vi "Dipper Fridge Resistance Measurement 2.0.vi"() -> ()   [LabVIEW 2011]
panel:
  in  "Lower critical\ntemperature":dbl
  in  "Upper critical\ntemperature":dbl
  out "x > y?":bool
  in  "critical temperature\n time delay":dbl
  out "error out":errorcluster
  in  "error in (no error)":errorcluster
  out "appended array 3":dbl[](array[numeric])
  out "appended array 2":dbl[](array[numeric])
  in  "General time delay":dbl
  out "appended array":dbl[](array[numeric])
  out "Temperature Vs Time":cluster{dbl[], dbl[]}(graph)
  out "Current Resistance":string
  in  "error in (no error) 3":errorcluster
  out "Current Temperature":string
  in  "Heater option":string
  out "Sample Vs. Temp":cluster{dbl[], dbl[]}(graph)
  out "Warning":string="Can't be smaller than 1 s"
  in  "Timer":bool caption="Reset"
  out "Time Elapsed":string
  in  "Save":bool
  out "var":i32
  out "Heater":bool
  in  "Heater":bool
  out "Boolean":bool
  in  "Power":bool
  in  "Date format (0)":enum16{"short", "long", "abbreviated"}(ring)
  in  "File Path":path
  out "current time":timestamp
  out "Data points":i32
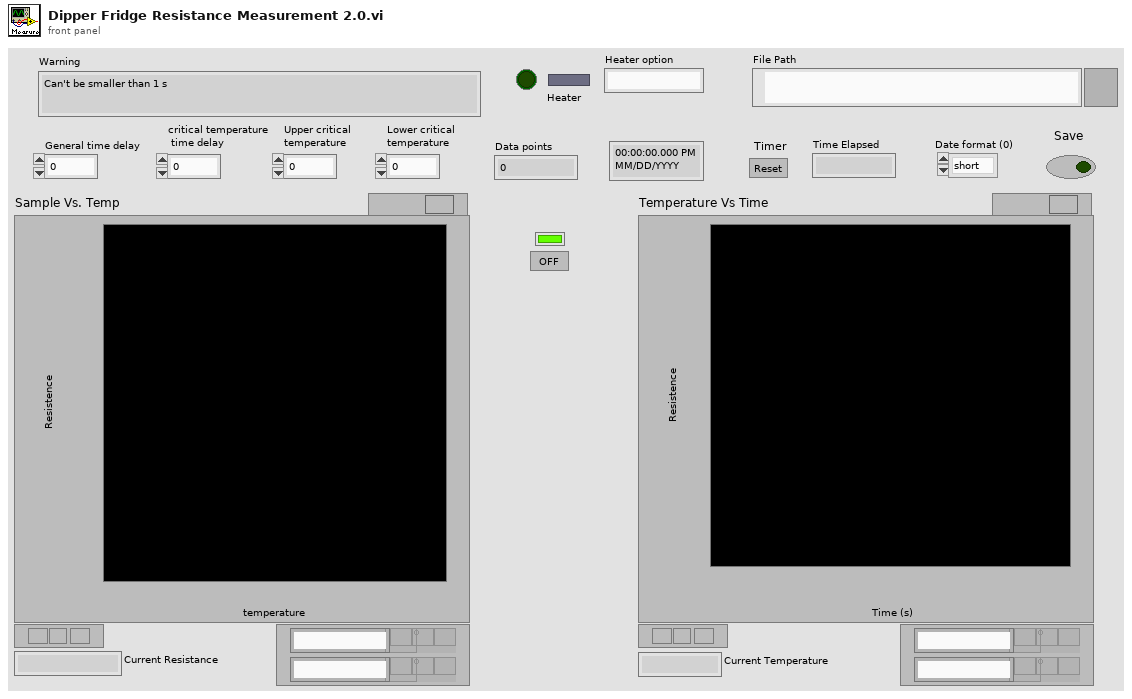
[diagram p1: front panel]
types:
  T1 = enum16{"open", "replace", "create", "open or create", "replace or create", "replace or create with confirmation"}
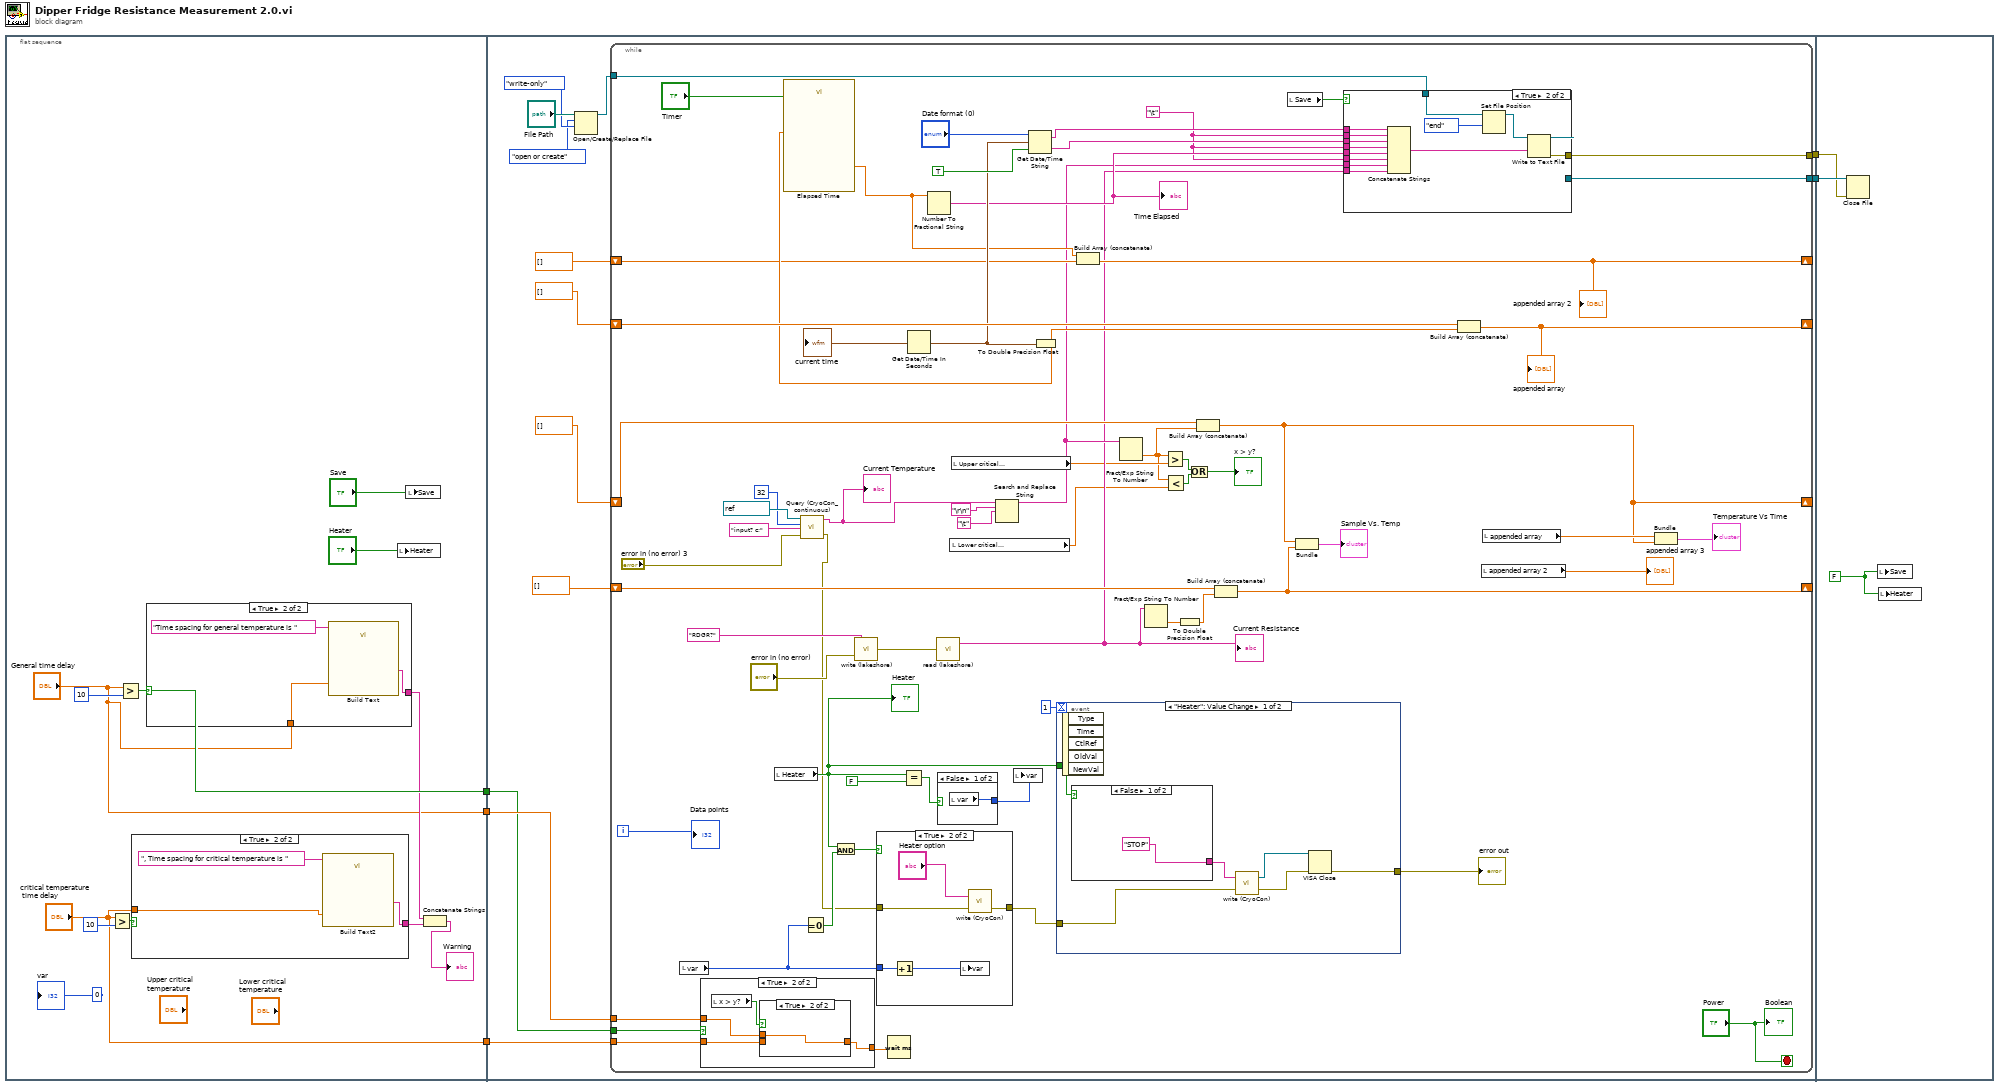
[diagram p0: block diagram]
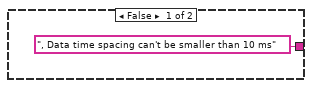
[diagram p2: hidden frame]
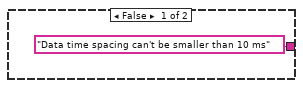
[diagram p3: hidden frame]
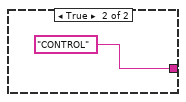
[diagram p4: hidden frame]
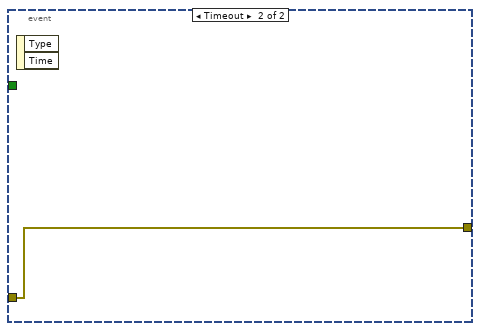
[diagram p5: hidden frame]
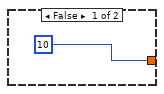
[diagram p6: hidden frame]
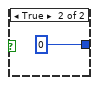
[diagram p8: hidden frame]
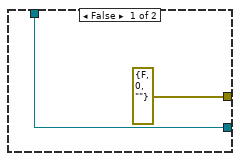
[diagram p10: hidden frame]
diagram:
  n1 = flat-sequence {
    tunnel: ["General time delay"] -> w5
    tunnel: [w13] -> w4
    tunnel: ["critical temperature\n time delay"] -> w1
    tunnel: w5 -> [w35]
    tunnel: w4 -> [w34]
    tunnel: [w28] -> w3
    tunnel: [w27] -> w2
    tunnel: w1 -> [w26]
    tunnel: w3 -> [w143]
    tunnel: w2 -> [w142]
    frame #0 {
      n2 = Greater?(x="critical temperature\n time delay", y=u32 10 ("x")) -> (0:w11:bool)
      n3 = Greater?(x="General time delay", y=u32 10 ("x")) -> (0:w13:bool)
      n4 = case shown="True" w11 {
        tunnel: [", Data time spacing can't be smaller than 10 ms" w21] -> w10
        tunnel: "critical temperature\n time delay" -> [_ w20]
        frame False {
        }
        frame True {
          n5 = call "Build Text2"("Beginning Text"=", Time spacing for critical temperature is ", "Y"=w20) -> ("Result"=w21:string)  [unwired: 12 in, 1 out]
        }
      }
      n6 = case shown="True" w13 {
        tunnel: "General time delay" -> [_ w24]
        tunnel: ["Data time spacing can't be smaller than 10 ms" w23] -> w9
        frame False {
        }
        frame True {
          n7 = call "Build Text"("Beginning Text"="Time spacing for general temperature is ", "Y"=w24) -> ("Result"=w23:string)  [unwired: 12 in, 1 out]
        }
      }
      n8 = local write "Heater"("Heater") -> ()
      n9 = local write "Save"("Save") -> ()
      n10 = Concatenate Strings(w9, w10) -> (→"Warning":string)
      "var" <- 0 ("var")
    }
    frame #1 {
      n11 = Open/Create/Replace File(file path (use dialog)="File Path", operation (0:open)=T1."open or create", access (0:read/write)=enum16{"read/write", "read-only", "write-only"}."write-only") -> (refnum out=w31:refnum<file>)  [unwired: 3 in, 2 out]
      n12 = while {
        shift-right: [w79] -> _
        shift-left: dbl[] [] -> [w99]
        shift-right: [w67] -> _
        shift-left: dbl[] [] -> [w97]
        shift-right: [w78] -> _
        shift-left: dbl[] [] -> [w83]
        tunnel: w35 -> [w80]
        tunnel: w34 -> [w81]
        shift-right: [w75] -> _
        shift-left: dbl[] [] -> [w76]
        tunnel: w31 -> [w54]
        tunnel: [w53] -> w28
        tunnel: [w52] -> w27
        tunnel: w26 -> [w45]
        i -> [w101]
        stop <- "Power" stop-if-true
        w57 = "\t"
        n13 = local read "var"() -> (w95:i32)
        n14 = case shown="True" w81 {
          tunnel: [10 w114] -> w82
          tunnel: w80 -> [_ w115]
          tunnel: w45 -> [_ w113]
          frame False {
          }
          frame True {
            n15 = local read "x > y?"() -> (w112:bool)
            n16 = case shown="True" w112 {
              tunnel: [w116 w117] -> w114
              tunnel: w115 -> [_ w117]
              tunnel: w113 -> [w116 _]
              frame False {
              }
              frame True {
              }
            }
          }
        }
        n17 = local read "Heater"() -> (w87:bool)
        "Heater" <- w87
        n18 = call "Query (CryoCon_continuous).vi"("error in (no error)"="error in (no error) 3", "write buffer"="input? c;", "byte count"=u32 32, "VISA resource name"=refnum<visa-resource-name> "COM3" ("VISA resource name 2")) -> ("error out"=w50:errorcluster, "read buffer"=w51:string)  [unwired: 1 out]
        "Current Temperature" <- w51
        n19 = Equal To 0?(x=w95) -> (x = 0?=w94:bool)
        n20 = And(x=w87, y=w94) -> (x .and. y?=w93:bool)
        n21 = call "write (lakeshore).vi"("error in (no error)"="error in (no error)", "write buffer"="RDGR?") -> ("error out"=w71:errorcluster)
        n22 = case shown="True" w93 {
          tunnel: [w120 w124] -> w92
          tunnel: w95 -> [_ w122]
          tunnel: w50 -> [w120 w123]
          frame False {
          }
          frame True {
            n23 = Increment(x=w122) -> (x+1=w121:i32)
            n24 = local write "var"(w121) -> ()
            n25 = call "write (CryoCon).vi"("error in (no error)"=w123, "write buffer"="Heater option") -> ("error out"=w124:errorcluster)  [unwired: 1 out]
          }
        }
        n26 = Wait (ms)(milliseconds to wait=w82) -> ()  [unwired: 1 out]
        n27 = Equal?(x=w87, y=FALSE ("Heater")) -> (x = y?=w89:bool)
        n28 = Get Date/Time In Seconds() -> (seconds since 1Jan1904=w86:timestamp)
        "current time" <- w86
        n29 = call "read (lakeshore).vi"("error in (no error)"=w71) -> ("read buffer"=w55:string)  [unwired: 1 out]
        "Current Resistance" <- w55
        n30 = case shown="False" w89 {
          tunnel: [w118 0] -> w88
          frame False {
            n31 = local read "var"() -> (w118:i32)
          }
          frame True {
          }
        }
        n32 = local read "Lower critical\ntemperature"() -> (w42:dbl)
        n33 = local read "Upper critical\ntemperature"() -> (w44:dbl)
        n34 = Search and Replace String(input string=w51, search string="\r\n", replace string="\t") -> (result string=w56:string)  [unwired: 5 in, 3 out]
        n35 = local write "var"(w88) -> ()
        n36 = Get Date/Time String(date format (0)="Date format (0)", seconds (now)=w86, want seconds? (F)=TRUE) -> (date string=w60:string, time string=w59:string)
        n37 = To Double Precision Float(number=w86) -> (double precision float=w85:dbl)
        n38 = call "Elapsed Time"("Reset"="Timer", "Set Start Time (s)"=w85) -> ("Elapsed Time (s)"=w77:dbl)  [unwired: 10 in, 7 out]
        n39 = Number To Fractional String(number=w77) -> (F-format string=w58:string)  [unwired: 3 in]
        "Time Elapsed" <- w58
        n40 = event shown="[0] \"Heater\": Value Change" {
          selector: _ -> [_ _]
          dyn-events: _ -> [_ _]
          timeout: 1 -> [_ _]
          tunnel: w92 -> [w106 w110]
          tunnel: w87 -> [w105 _]
          tunnel: [w102 w110] -> w61
          event "Heater": Value Change {
            n41 = event-data() -> ()  [unwired: 1 in, 5 out]
            n42 = case shown="False" w105 {
              tunnel: ["STOP" ("write buffer") "CONTROL" ("write buffer")] -> w107
              frame False {
              }
              frame True {
              }
            }
            n43 = call "write (CryoCon).vi"("error in (no error)"=w106, "write buffer"=w107) -> ("error out"=w103:errorcluster, "VISA resource name out"=w104:refnum<visa-resource-name>)
            n44 = VISA Close(VISA resource name=w104, error in (no error)=w103) -> (error out=w102:errorcluster)
          }
          event Timeout {
            n45 = event-data() -> ()  [unwired: 1 in, 2 out]
          }
        }
        "error out" <- w61
        n46 = Build Array (concatenate)(w77, w76) -> (w75:dbl[])
        "appended array 2" <- w75
        n47 = Fract/Exp String To Number(string=w56) -> (number=w43:dbl)  [unwired: 3 in, 1 out]
        n48 = Fract/Exp String To Number(string=w55) -> (number=w65:dbl)  [unwired: 3 in, 1 out]
        n49 = Greater?(x=w43, y=w44) -> (0:w40:bool)
        n50 = Less?(x=w43, y=w42) -> (x < y?=w41:bool)
        n51 = To Double Precision Float(number=w65) -> (double precision float=w69:dbl)
        n52 = Or(x=w40, y=w41) -> (x .or. y?=→"x > y?":bool)
        n53 = Build Array (concatenate)(w97, w43) -> (w67:dbl[])
        n54 = Build Array (concatenate)(w83, w69) -> (w78:dbl[])
        n55 = local read "Save"() -> (w91:bool)
        n56 = Bundle(w67, w78) -> (→"Sample Vs. Temp":cluster{dbl[], dbl[]})  [unwired: 1 in]
        n57 = case shown="True" w91 {
          tunnel: w56 -> [_ w133]
          tunnel: w60 -> [_ w139]
          tunnel: w57 -> [_ w138]
          tunnel: w59 -> [_ w137]
          tunnel: w57 -> [_ w136]
          tunnel: w58 -> [_ w135]
          tunnel: w57 -> [_ w134]
          tunnel: w55 -> [_ w132]
          tunnel: w54 -> [w127 w131]
          tunnel: [w127 w129] -> w53
          tunnel: [errorcluster {"status"=FALSE, "code"=0, "source"=""} ("error out") w128] -> w52
          frame False {
          }
          frame True {
            n58 = Concatenate Strings(w139, w138, w137, w136, w135, w134, w133, w132) -> (w130:string)
            n59 = Set File Position(refnum=w131, from (0:start)=enum16{"start", "end", "current"}."end") -> (refnum out=w140:refnum<file>)  [unwired: 2 in, 1 out]
            n60 = Write to Text File(file (use dialog)=w140, text=w130) -> (refnum out=w129:refnum<file>, error out=w128:errorcluster)  [unwired: 2 in, 1 out]
          }
        }
        n61 = Build Array (concatenate)(w99, w85) -> (w79:dbl[])
        "appended array" <- w79
        n62 = local read "appended array 2"() -> (→"appended array 3":dbl[])
        n63 = local read "appended array"() -> (w73:dbl[])
        n64 = Bundle("appended array"=w73, w67) -> (→"Temperature Vs Time":cluster{"appended array":dbl[], dbl[]})  [unwired: 1 in]
        "Data points" <- w101
        "Boolean" <- "Power"
      }
    }
    frame #2 {
      w144 = FALSE ("Save")
      n65 = Close File(refnum=w143, error in=w142) -> ()  [unwired: 2 out]
      n66 = local write "Save"(w144) -> ()
      n67 = local write "Heater"(w144) -> ()
    }
  }
